vi "Motic Get Frame.vi"(8 "error in (no error)":errorcluster, 10 "image buffer in":u8[](array[numeric]), 11 "camera":i32) -> (0 "error out":errorcluster, 2 "image buffer out":u8[](array[numeric]), 3 "camera out":i32, 5 "timestamp out":u32)   [LabVIEW 2012, in "MoticApi.lvlib"]
doc: "MOTICAPI bool Motic_GetFrame(MUCam_Handle camera, unsigned char *buf, unsigned long *ts);"
uses:
  MoticApi.lvlib
  MoticApi.dll
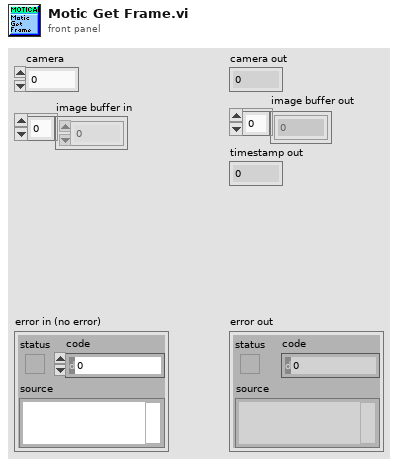
[diagram p1: front panel]
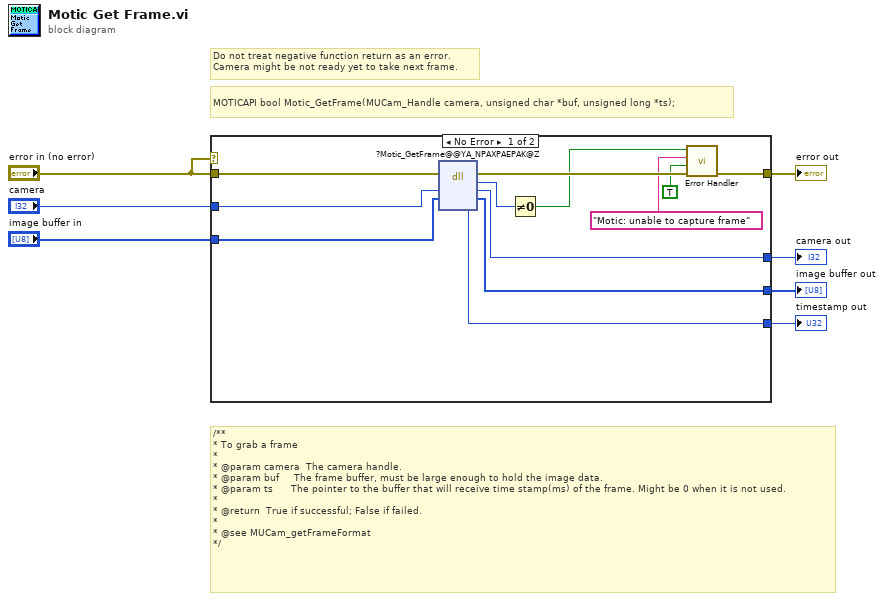
[diagram p0: block diagram]
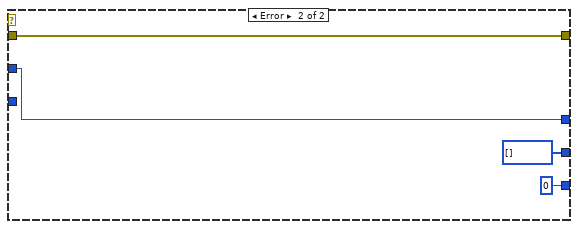
[diagram p2: hidden frame]
diagram:
  # "/**\n* To grab a frame\n*\n* @param camera  The camera handle.\n* @param buf     The frame buffer, must be large enough to hold the image data.\n* @param ts      The pointer to the buffer that will receive time stamp(ms) of the frame. Might be 0 when it is not used.\n*\n* @return  True if successful; False if failed.\n*\n* @see MUCam_getFrameFormat\n*/"
  # "Do not treat negative function return as an error.\nCamera might be not ready yet to take next frame."
  # "MOTICAPI bool Motic_GetFrame(MUCam_Handle camera, unsigned char *buf, unsigned long *ts);"
  n1 = case shown="No Error" "error in (no error)" {
    tunnel: "camera" -> [w18 w22]
    tunnel: [w17 w22] -> w6
    tunnel: [w16 u8[] [] ("buf")] -> w5
    tunnel: "error in (no error)" -> [w15 w23]
    tunnel: [w14 u32 0 ("ts")] -> w4
    tunnel: [w10 w23] -> w3
    tunnel: "image buffer in" -> [w8 _]
    frame No Error {
      n2 = dll-call lib="C:/Users/TTS-Digital/Desktop/MoticApi/MoticApi_git/MoticApi/MoticApi.*" fn="?Motic_GetFrame@@YA_NPAXPAEPAK@Z"(error in=w15, "camera"=w18, "buf"=w8) -> (error out=w13:errorcluster, "return type"=w19:u8, "camera"=w17:i32, "buf"=w16:u8[], "ts"=w14:u32)  [unwired: 3 in, 1 out]
      n3 = Not Equal To 0?(x=w19) -> (x != 0?=w12:bool)
      n4 = call "Error Handler.vi"("error in (no error)"=w13, "Is warning?"=TRUE, "Error message"="Motic: unable to capture frame" ("error message (\"\")"), "Function return"=w12) -> ("error out"=w10:errorcluster)  [unwired: 7 in]
    }
    frame Error {
    }
  }
  "camera out" <- w6
  "image buffer out" <- w5
  "timestamp out" <- w4
  "error out" <- w3
